vi "QPMX Set Path.vi"(8 "error in":errorcluster, 10 "path":string, 11 "QPMX ssn":T1={"visa"="", "switch mode"=enum."Switched by TWM", "sequence"=[], "timing delays"=[], "polarity"=enum."Positive", "ss delay (s)"=2.0} {"ss delay (s)" min=0.0 step=1.0; "timing delays" min=1 max=255 step=1}) -> (0 "error out":errorcluster, 2 "Time delay (s)":dbl, 3 "QPMX ssn out":T1={"visa"="", "switch mode"=enum."Switched by TWM", "sequence"=[], "timing delays"=[], "polarity"=enum."Positive", "ss delay (s)"=2.0} {"ss delay (s)" min=0.0 step=1.0; "timing delays" min=1 max=255 step=1})   [LabVIEW 2020]
doc: "Wrapper layer between TWM and QuPMXdriver. Initialize multiplexer."
uses:
  Generic COM/QPMX Session.ctl
  QPMX switch mode.ctl
  QPMX polarity.ctl
  QuPMXLabVIEWdriver/QuPMXdriver.lvlib
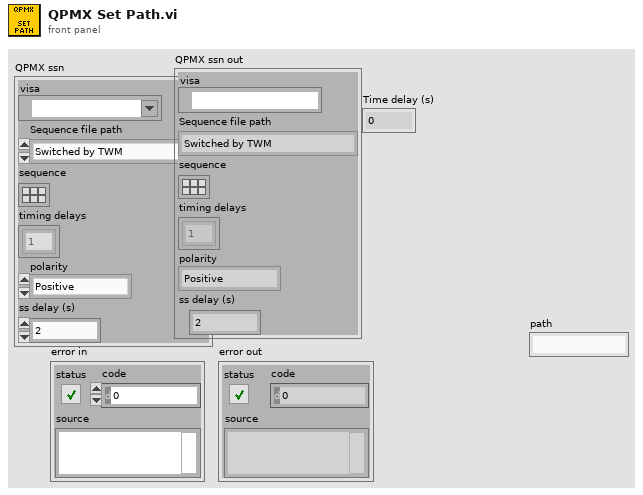
[diagram p1: front panel]
types:
  T1 = typedef "QPMX Session.ctl" = cluster{"visa":refnum<visa-resource-name>, "switch mode":T2, "sequence":bool[][], "timing delays":u32[], "polarity":T3, "ss delay (s)":dbl}
  T2 = typedef "QPMX switch mode.ctl" = enum16{"Switched by TWM", "Switched by external clock", "Switched by internal clock"}
  T3 = typedef "QPMX polarity.ctl" = enum16{"Positive", "Negative"}
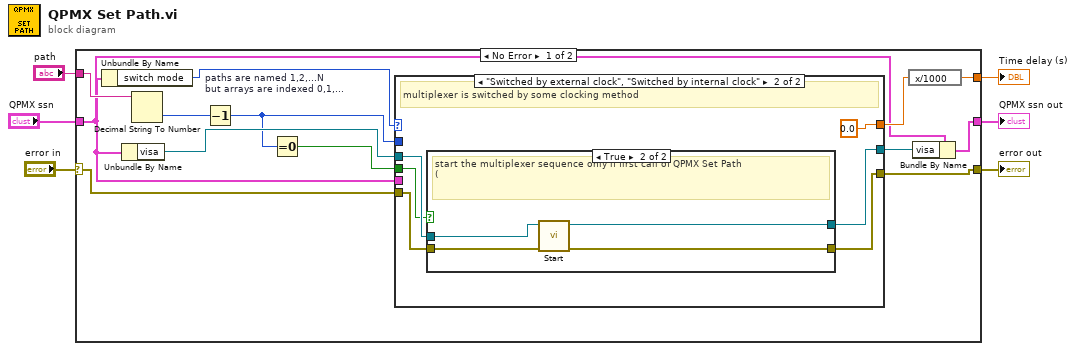
[diagram p0: block diagram]
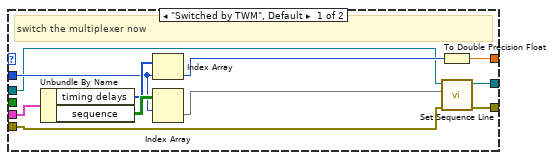
[diagram p2: hidden frame]
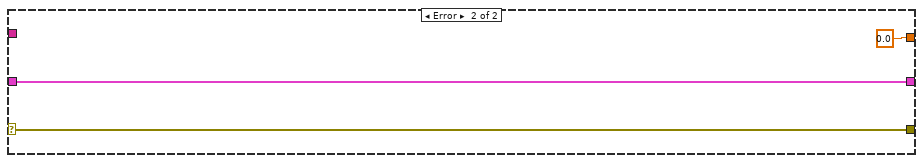
[diagram p4: hidden frame]
diagram:
  n1 = case shown="No Error" "error in" {
    selector: "error in" -> [w17 w45]
    tunnel: [w16 w45] -> w5
    tunnel: "QPMX ssn" -> [w10 w44]
    tunnel: [w19 w44] -> w3
    tunnel: "path" -> [w18 _]
    tunnel: [w14 0.0 ("Numeric")] -> w1
    frame No Error {
      n2 = Unbundle By Name(w10) -> ("switch mode"=w12:T2)
      n3 = Unbundle By Name(w10) -> ("visa"=w11:refnum<visa-resource-name>)
      n4 = Decimal String To Number(string=w18) -> (number=w9:i32)  [unwired: 2 in, 1 out]
      n5 = Decrement "paths are named 1,2,...N\nbut arrays are indexed 0,1,..."(x=w9) -> (x-1=w7:i32)
      n6 = Equal To 0?(x=w7) -> (x = 0?=w8:bool)
      n7 = case shown="\"Switched by external clock\", \"Switched by internal clock\"" w12 {
        tunnel: w17 -> [w29 w35]
        tunnel: [w26 w34] -> w16
        tunnel: [w25 w33] -> w15
        tunnel: [w23 0.0] -> w13
        tunnel: w7 -> [w22 _]
        tunnel: w10 -> [w21 _]
        tunnel: w11 -> [w20 w36]
        tunnel: w8 -> [_ w31]
        frame "Switched by TWM", Default {
          # "switch the multiplexer now"
          n8 = Unbundle By Name(w21) -> ("timing delays"=w27:u32[], "sequence"=w30:bool[][])
          n9 = Index Array(array=w27, index=w22) -> (element=w24:u32)
          n10 = Index Array(array=w30, index (row)=w22) -> (element=w28:bool[])  [unwired: 1 in]
          n11 = To Double Precision Float(number=w24) -> (double precision float=w23:dbl)
          n12 = call "Set Sequence Line.vi"("error in (no error)"=w29, "Sequence Line"=w28, "VISA resource name"=w20) -> ("error out"=w26:errorcluster, "VISA resource name out"=w25:refnum<visa-resource-name>)  [unwired: 7 in]
        }
        frame "Switched by external clock", "Switched by internal clock" {
          # "multiplexer is switched by some clocking method"
          n13 = case shown="True" w31 {
            tunnel: w36 -> [w38 w42]
            tunnel: w35 -> [w37 w41]
            tunnel: [w37 w40] -> w34
            tunnel: [w38 w39] -> w33
            frame False {
              # "on second and other calls of this vi do nothing,\nmultiplexer is already running a sequence"
            }
            frame True {
              # "start the multiplexer sequence only if first call of QPMX Set Path\n("
              n14 = call "Start.vi"("error in (no error)"=w41, "VISA resource name"=w42) -> ("error out"=w40:errorcluster, "VISA resource name out"=w39:refnum<visa-resource-name>)  [unwired: 8 in]
            }
          }
        }
      }
      n15 = expression code="x/1000"(w13) -> (w14:dbl)
      n16 = Bundle By Name(cluster=w10, "visa"=w15) -> (w19:T1)
    }
    frame Error {
    }
  }
  "error out" <- w5
  "QPMX ssn out" <- w3
  "Time delay (s)" <- w1
